vi "HCC Agilent Tester.vi"() -> ()   [LabVIEW 2016]
uses:
  Agilent 34970.lvlib
panel:
  out "Clean Analog Scan List":string
  out "Instrument IDN":string
  in  "VISA Resource Name":refnum<visa-resource-name>
  in  "stop":bool
  in  "Disable Channel = True":bool[](array[boolean])
  out "Current":dbl[](array[numeric])
  out "Raw Data (Scaled)":dbl[](array[numeric]) format="%.2f"
  out "Unsorted Data":dbl[](array[numeric]) format="%.2f"
  out "read buffer":string
  in  "Channel List":string="(1_0_L11Current)101,(1_0_L11Current)102,(1_0_L11Current)103"
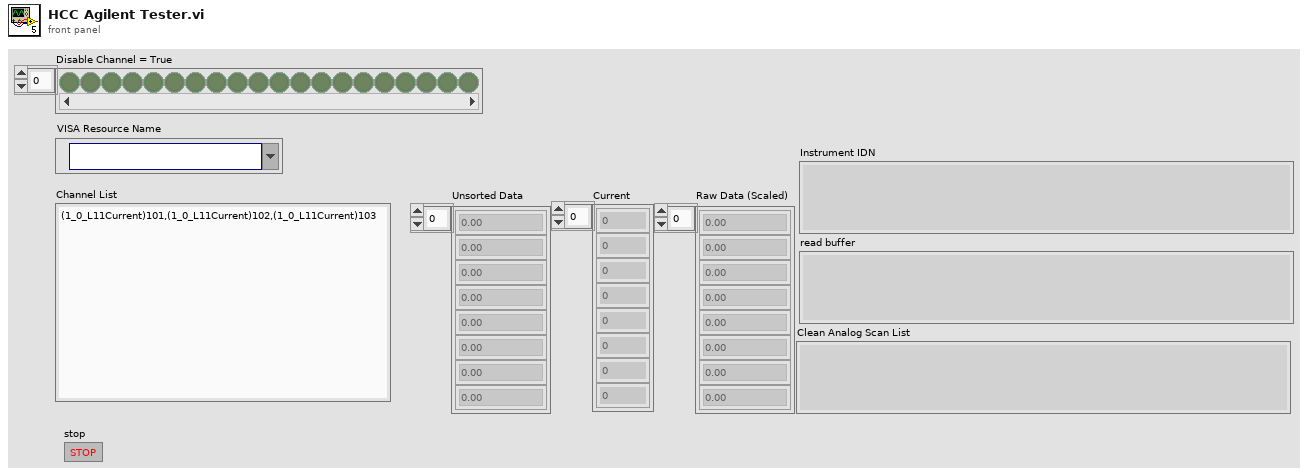
[diagram p1: front panel]
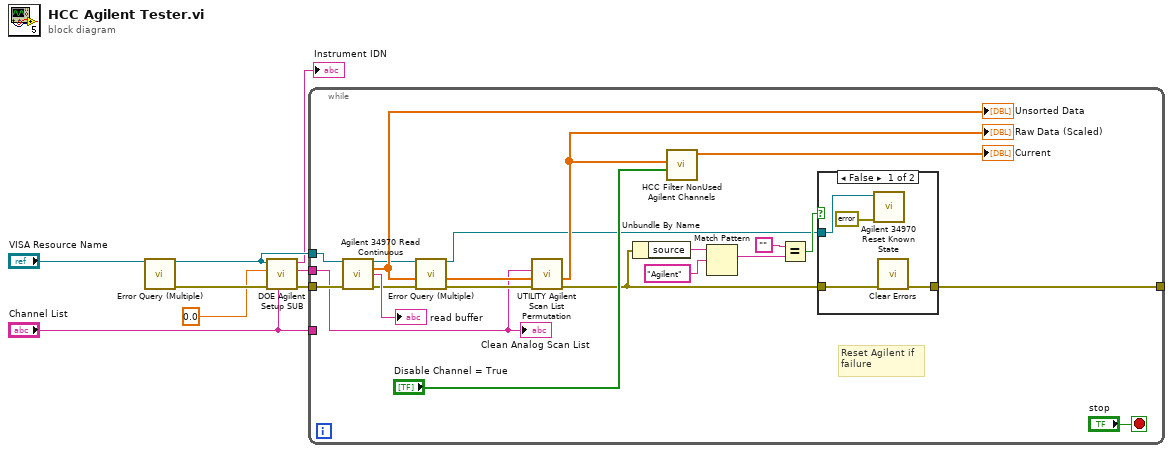
[diagram p0: block diagram]
diagram:
  n1 = call "Error Query (Multiple).vi"("VISA Resource Name"="VISA Resource Name") -> ("VISA Resource Name Out"=w5:refnum<visa-resource-name>, "error out"=w7:errorcluster)  [unwired: 11 in, 2 out]
  n2 = call "DOE Agilent Setup SUB.vi"("Analog Channels-List"="Channel List", "error in (no error)"=w7, "Agilent Gain"=0.0, "VISA Refnum in"=w5) -> ("error out"=w6:errorcluster, "Clean Analog Scan List"=w3:string, "Instrument IDN"=→"Instrument IDN":string)  [unwired: 5 in]
  n3 = while {
    tunnel: w6 -> [w18]
    tunnel: w5 -> [w17]
    tunnel: [w16] -> _
    tunnel: "Channel List" -> [_]
    tunnel: w3 -> [w9]
    stop <- "stop" stop-if-true
    # "Reset Agilent if \nfailure"
    n4 = call "Agilent 34970 Read Continuous.vi"("VISA Resource Name"=w17, "error in (no error)"=w18) -> ("VISA resource name out"=w10:refnum<visa-resource-name>, "Output Array"=w20:dbl[], "read buffer"=→"read buffer":string, "error out"=w14:errorcluster)  [unwired: 10 in]
    "Unsorted Data" <- w20
    n5 = call "Error Query (Multiple).vi"("VISA Resource Name"=w10, "error in (no error)"=w14) -> ("VISA Resource Name Out"=w11:refnum<visa-resource-name>, "error out"=w13:errorcluster)  [unwired: 10 in, 2 out]
    n6 = call "UTILITY Agilent Scan List Permutation.vi"("Error In"=w13, "Input Data Array"=w20, "Agilent Scan List"=w9) -> ("Error Out"=w12:errorcluster, "Output Data Permutation"=w26:dbl[])  [unwired: 6 in, 1 out]
    "Raw Data (Scaled)" <- w26
    n7 = Unbundle By Name(w12) -> ("source"=w25:string)
    n8 = call "HCC Filter NonUsed Agilent Channels.vi"("Disable Channel = True"="Disable Channel = True", "Input Current"=w26) -> ("Output Current"=→"Current":dbl[])  [unwired: 7 in, 2 out]
    n9 = Match Pattern(string=w25, regular expression="Agilent") -> (match substring=w21:string)  [unwired: 1 in, 3 out]
    n10 = Equal?(x="", y=w21) -> (x = y?=w23:bool)
    n11 = case shown="False" w23 {
      tunnel: w12 -> [w30 w33]
      tunnel: [w29 w33] -> w16
      tunnel: w11 -> [w31 _]
      frame False {
        n12 = call "Agilent 34970 Reset Known State.vi"("Error In"=errorcluster {"status"=TRUE, "code"=0, "source"=""}, "VISA Refnum in"=w31) -> ()  [unwired: 9 in, 1 out]
        n13 = call <vilib>:"Clear Errors.vi"("error in (no error)"=w30) -> ("error out"=w29:errorcluster)  [unwired: 5 in, 1 out]
      }
      frame True {
      }
    }
    "Clean Analog Scan List" <- w9
  }
